vi "ArchViewer.vi"() -> ()   [LabVIEW 2010]
doc: "Use this template to create an application that executes until you click the Stop button. Unlike the Single Loop Application VI that uses polling, this VI uses the Event structure."
uses:
  <vilib>/addons/database/Connection.llb/DB Tools Open Connec (Path).vi
  <vilib>/addons/database/NI_Database_API.lvlib
panel:
  in  "save":bool
  out "Message":string
  out "ObjProp":string[][](table)
  in  "ViewMode":enum32{"Графики", "Тренды", "SQL"}(tab)=enum."Тренды"
  out "reason":string caption="Описание"
  in  "DateAndTime":u16(ring) caption="Дата и Время" items=["2010-03-20 19:57:10", "2010-03-20 19:58:10", "2010-03-20 19:59:11", "2010-03-20 20:00:11", "2010-03-20 20:01:12", "2010-03-20 20:02:12", "2010-03-20 20:03:13"]
  out "Waveform Graph":cluster{sgl, sgl, sgl[]}[](graph)
  in  "CurvesName":i32(ring) caption="Сигнал (Тип сигнала)" items=["Q(wt)max"=400301, "Q(wt)mean"=500301, "Q(R)"=300301, "I(R)"=100301, "N(Q)"=200301]
  out "XY Graph":cluster{timestamp[], sgl[]}(graph)
  in  "T final":timestamp caption="Конец интервала"
  in  "T start":timestamp caption="Начало"
  in  "SigName":u16(ring) caption="Сигнал" items=["In(Напряжение/Ток)"=302, "Out(Напряжение/Ток)"=301]
  in  "Numeric":i32 min=0 max=9
  in  "Execute":bool
  out "Data":string[][](table) caption="Данные"
  in  "Query":string caption="Запрос"
  in  "Tables":i32(listbox) caption="Таблицы"
  in  "Object":u16(ring) caption="Объект" items=["test1", "К-19 Тц", "Безымянный", "test2"]
  in  "stop":bool
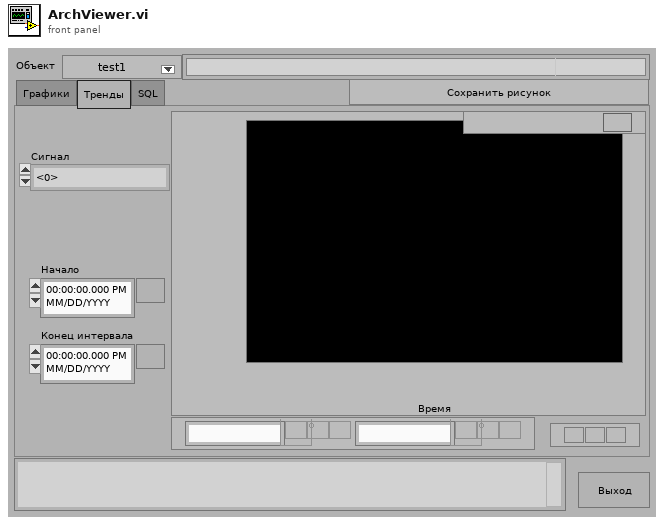
[diagram p1: front panel]
types:
  T1 = typedef "NI_Database_API.lvlib/Conn ObjectReference.ctl" = refnum<k1>
  T2 = cluster{"recordset data[0]":variant, "recordset data[1]":variant}
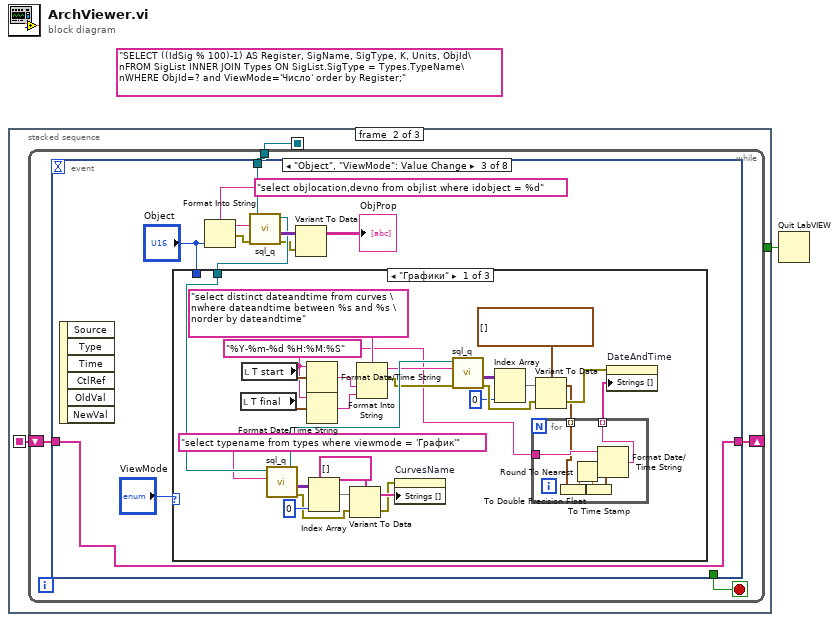
[diagram p0: block diagram]
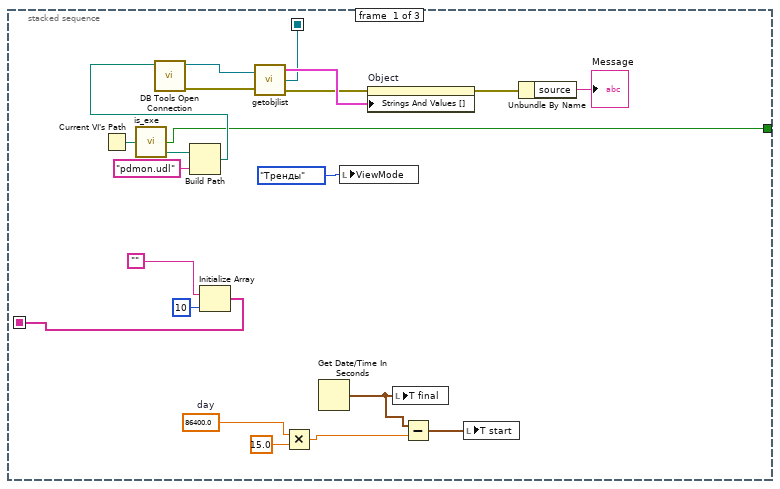
[diagram p2: hidden frame]
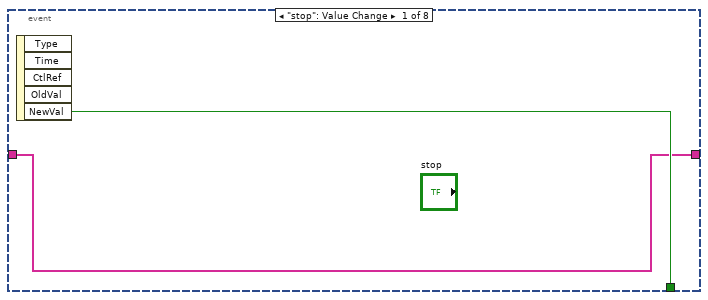
[diagram p3: hidden frame]
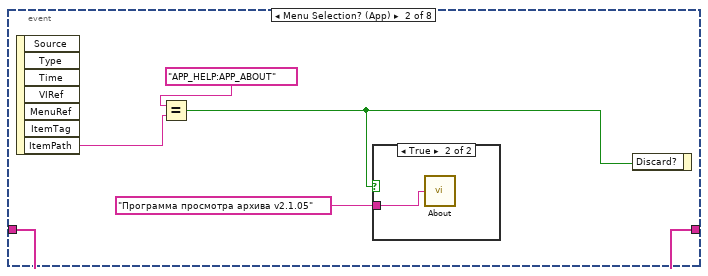
[diagram p4: hidden frame]
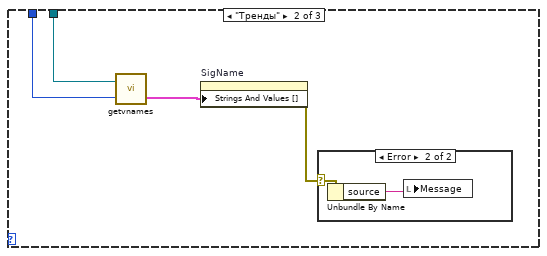
[diagram p6: hidden frame]
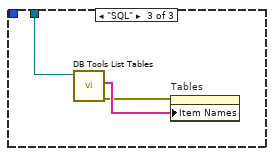
[diagram p8: hidden frame]
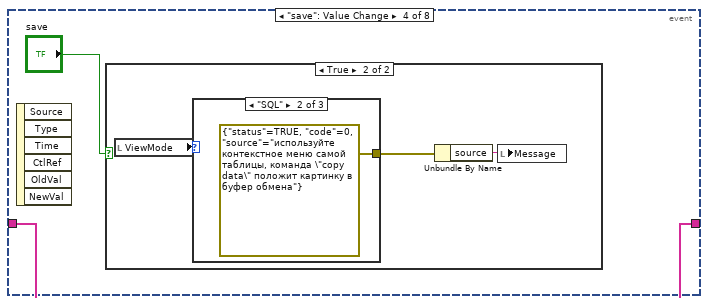
[diagram p9: hidden frame]
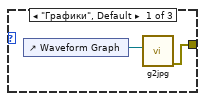
[diagram p11: hidden frame]
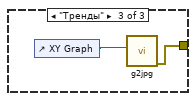
[diagram p12: hidden frame]
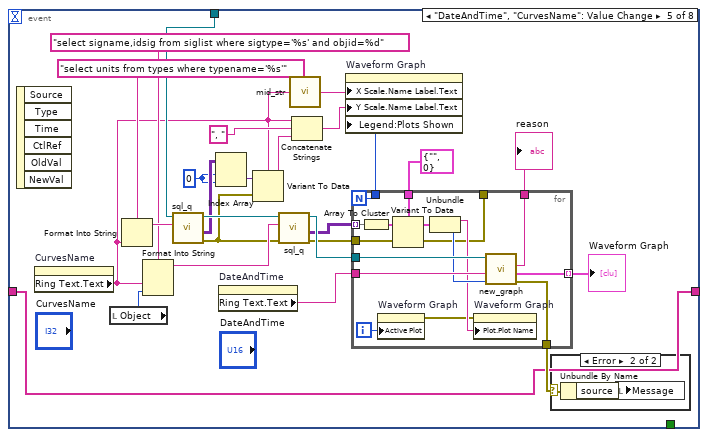
[diagram p13: hidden frame]
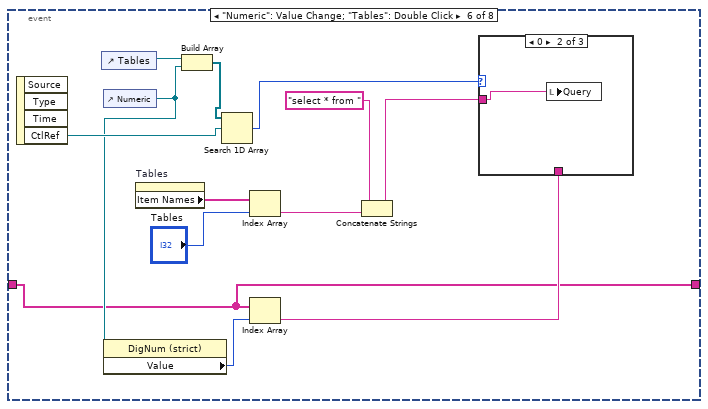
[diagram p15: hidden frame]
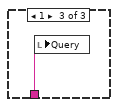
[diagram p17: hidden frame]
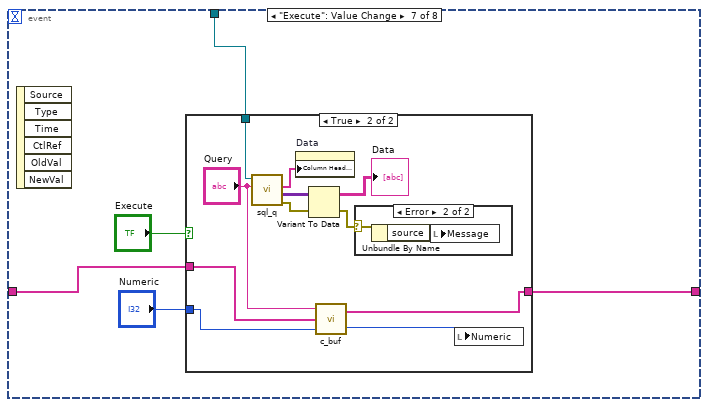
[diagram p18: hidden frame]
diagram:
  (unwired) "SELECT ((IdSig % 100)-1) AS Register, SigName, SigType, K, Units, ObjId\nFROM SigList INNER JOIN Types ON SigList.SigType = Types.TypeName\nWHERE ObjId=? and ViewMode='Число' order by Register;"
  n1 = stacked-sequence {
    seq-local: [w18 _ _] -> [_ w24 w189]
    seq-local: [w3 _ _] -> [_ w23 _]
    tunnel: [w2 _ _] -> w1
    frame #0 {
      w8 = 86400.0  # day
      n2 = Current VI's Path() -> (path=w14:path)
      n3 = call "is_exe.vi"("path"=w14) -> ("actual path"=w13:path, "exe?"=w2:bool)  [unwired: 2 in, 1 out]
      n4 = Build Path(base path=w13, name or relative path="pdmon.udl") -> (appended path=w11:path)
      n5 = call-poly <vilib>:"DB Tools Open Connection.vi"("connection information"=w11) -> ("error out"=w19:errorcluster, "connection reference"=w20:T1)  [unwired: 7 in]
      n6 = Initialize Array("", 10 ("dimension size")) -> (w3:string[])
      n7 = call "getobjlist.vi"("connection"=w20, "error in"=w19) -> ("StringsAndValues[]"=w22:cluster{"String":string, "Value":u16}[], "connection out"=w18:T1, "error out"=w21:errorcluster)
      n8 = Multiply(x=w8, y=15.0) -> (x*y=w7:dbl)
      n9 = Get Date/Time In Seconds() -> (seconds since 1Jan1904=w10:timestamp)
      n10 = local write "ViewMode"(enum32{"Графики", "Тренды", "SQL"}."Тренды" ("ViewMode")) -> ()
      n11 = property on="Object" class="Ring (strict)"(error in=w21, "Strings And Values []"=w22) -> (error out=w17:errorcluster)  [unwired: 1 in, 1 out]
      n12 = local write "T final"(w10) -> ()
      n13 = Subtract(x=w10, y=w7) -> (x-y=w9:timestamp)
      n14 = local write "T start"(w9) -> ()
      n15 = Unbundle By Name(w17) -> ("source"=→"Message":string)
    }
    frame #1 {
      n16 = while {
        tunnel: w24 -> [w27]
        shift-right: [w26] -> _
        shift-left: w23 -> [w25]
        stop <- w28 stop-if-true
        n17 = event shown="[2] \"Object\", \"ViewMode\": Value Change" {
          selector: _ -> [_ _ _ _ _ _ _ _]
          dyn-events: _ -> [_ _ _ _ _ _ _ _]
          timeout: _ -> [_ _ _ _ _ _ _ _]
          tunnel: [w30 _ _ _ _ _ _ _] -> w28
          tunnel: w27 -> [_ _ w43 _ w112 _ w162 w186]
          tunnel: [w29 w35 w37 w89 w99 w143 w159 w178] -> w26
          tunnel: w25 -> [w29 w35 w37 w89 w99 w143 w158 w178]
          event "stop": Value Change {
            n18 = event-data() -> ("NewVal"=w30:bool)  [unwired: 1 in, 4 out]
          }
          event Menu Selection? (App) {
            n19 = event-data() -> ("ItemPath"=w33:string)  [unwired: 1 in, 6 out]
            n20 = Equal?(x="APP_HELP:APP_ABOUT", y=w33) -> (x = y?=w32:bool)
            n21 = case shown="True" w32 {
              tunnel: "Программа просмотра архива v2.1.05" -> [_ w36]
              frame False {
              }
              frame True {
                n22 = call "About.vi"("Revision Number"=w36) -> ()
              }
            }
            n23 = event-data("Discard?"=w32) -> ()  [unwired: 1 in, 1 out]
          }
          event "Object", "ViewMode": Value Change {
            n24 = event-data() -> ()  [unwired: 1 in, 6 out]
            n25 = Format Into String(format string="select objlocation,devno from objlist where idobject = %d", "Object") -> (resulting string=w46:string, error out=w39:errorcluster)  [unwired: 2 in]
            n26 = call "sql_q.vi"("error in"=w39, "SQL query"=w46, "connect ref"=w43) -> ("error out"=w41:errorcluster, "recordset data"=w45:variant[][], "conn ref out"=w42:T1)  [unwired: 1 in, 1 out]
            n27 = case shown="\"Графики\"" "ViewMode" {
              tunnel: w42 -> [w73 w82 w88]
              tunnel: "Object" -> [_ w81 _]
              frame "Графики" {
                w49 = "%Y-%m-%d %H:%M:%S" ("time format string (%c)")
                n28 = local read "T final"() -> (w60:timestamp)
                n29 = local read "T start"() -> (w61:timestamp)
                n30 = call "sql_q.vi"("SQL query"="select typename from types where viewmode = 'График'", "connect ref"=w73) -> ("error out"=w66:errorcluster, "recordset data"=w71:variant[][], "conn ref out"=w55:T1)  [unwired: 2 in, 1 out]
                n31 = Format Date/Time String(time format string (%c)=w49, seconds (now)=w61) -> (date/time string=w63:string)  [unwired: 1 in]
                n32 = Format Date/Time String(time format string (%c)=w49, seconds (now)=w60) -> (date/time string=w64:string)  [unwired: 1 in]
                n33 = Index Array(array=w71, index (col)=0 ("disabled index (col)")) -> (element=w68:variant[])  [unwired: 1 in]
                n34 = Variant To Data(error in=w66, Variant=w68, type=string[] [] ("Strings []")) -> (error out=w65:errorcluster, data=w70:string[])
                n35 = Format Into String(format string="select distinct dateandtime from curves \nwhere dateandtime between %s and %s \norder by dateandtime", w63, w64) -> (resulting string=w54:string, error out=w53:errorcluster)  [unwired: 2 in]
                n36 = property on="CurvesName" class="Ring (strict)"(error in=w65, "Strings []"=w70) -> ()  [unwired: 1 in, 2 out]
                n37 = call "sql_q.vi"("error in"=w53, "SQL query"=w54, "connect ref"=w55) -> ("error out"=w59:errorcluster, "recordset data"=w56:variant[][])  [unwired: 1 in, 2 out]
                n38 = Index Array(array=w56, index (col)=0 ("disabled index (col)")) -> (element=w57:variant[])  [unwired: 1 in]
                n39 = Variant To Data(error in=w59, Variant=w57, type=timestamp[] [] ("Strings []")) -> (error out=w52:errorcluster, data=w51:timestamp[])
                n40 = for {
                  tunnel: w51 -> [w74] mode=indexing
                  tunnel: [w79] -> w50 mode=indexing
                  tunnel: w49 -> [w78]
                  n41 = To Double Precision Float(number=w74) -> (double precision float=w76:dbl)
                  n42 = Round To Nearest(number=w76) -> (nearest integer value=w75:dbl)
                  n43 = To Time Stamp(1:w75) -> (0:w77:timestamp)
                  n44 = Format Date/Time String(time format string (%c)=w78, seconds (now)=w77) -> (date/time string=w79:string)  [unwired: 1 in]
                }
                n45 = property on="DateAndTime" class="Ring (strict)"(error in=w52, "Strings []"=w50) -> ()  [unwired: 1 in, 2 out]
              }
              frame "Тренды" {
                n46 = call "getvnames.vi"("Object"=w81, "connection reference in"=w82) -> ("StringsAndValues[]"=w83:cluster{"String":string, "Value":u16}[])  [unwired: 1 out]
                n47 = property on="SigName" class="Ring (strict)"("Strings And Values []"=w83) -> (error out=w80:errorcluster)  [unwired: 2 in, 1 out]
                n48 = case shown="Error" w80 {
                  selector: w80 -> [_ w85]
                  frame No Error {
                  }
                  frame Error {
                    n49 = Unbundle By Name(w85) -> ("source"=w84:string)
                    n50 = local write "Message"(w84) -> ()
                  }
                }
              }
              frame "SQL" {
                n51 = call <vilib>:"DB Tools List Tables.vi"("connection reference"=w88) -> ("error out"=w86:errorcluster, "tables"=w87:string[])  [unwired: 4 in, 1 out]
                n52 = property on="Tables" class="LstBox (strict)"(error in=w86, "Item Names"=w87) -> ()  [unwired: 1 in, 2 out]
              }
            }
            n53 = Variant To Data(error in=w41, Variant=w45) -> (data=→"ObjProp":string[][])  [unwired: 1 in, 1 out]
          }
          event "save": Value Change {
            n54 = event-data() -> ()  [unwired: 1 in, 6 out]
            n55 = case shown="True" "save" {
              frame False {
              }
              frame True {
                n56 = local read "ViewMode"() -> (w93:enum32{"Графики", "Тренды", "SQL"})
                n57 = case shown="\"SQL\"" w93 {
                  tunnel: [w94 errorcluster {"status"=TRUE, "code"=0, "source"="используйте контекстное меню самой таблицы, команда \"copy data\" положит картинку в буфер обмена"} ("error out") w97] -> w92
                  frame "Графики", Default {
                    n58 = control-ref of="Waveform Graph"() -> (w95:refnum<vi>)
                    n59 = call "g2jpg.vi"("WG"=w95) -> ("error out"=w94:errorcluster)  [unwired: 5 in, 1 out]
                  }
                  frame "SQL" {
                  }
                  frame "Тренды" {
                    n60 = control-ref of="XY Graph"() -> (w98:refnum<vi>)
                    n61 = call "g2jpg.vi"("WG"=w98) -> ("error out"=w97:errorcluster)  [unwired: 5 in, 1 out]
                  }
                }
                n62 = Unbundle By Name(w92) -> ("source"=w91:string)
                n63 = local write "Message"(w91) -> ()
              }
            }
          }
          event "DateAndTime", "CurvesName": Value Change {
            w108 = 0
            n64 = event-data() -> ()  [unwired: 1 in, 6 out]
            n65 = property on="CurvesName" class="Ring (strict)"() -> ("Ring Text.Text"=w100:string)  [unwired: 2 in, 2 out]
            n66 = local read "Object"() -> (w120:u16)
            n67 = Format Into String(format string="select units from types where typename='%s'", w100) -> (resulting string=w113:string)  [unwired: 2 in, 1 out]
            n68 = Format Into String(format string="select signame,idsig from siglist where sigtype='%s' and objid=%d" ("regular expression (\"\")"), w100, w120) -> (resulting string=w121:string)  [unwired: 2 in, 1 out]
            n69 = call "sql_q.vi"("SQL query"=w113, "connect ref"=w112) -> ("error out"=w105:errorcluster, "recordset data"=w109:variant[][], "conn ref out"=w111:T1)  [unwired: 2 in, 1 out]
            n70 = Index Array(array=w109, index (row)=w108, index (col)=w108) -> (element=w107:variant)
            n71 = property on="DateAndTime" class="Ring (strict)"() -> ("Ring Text.Text"=w124:string)  [unwired: 2 in, 2 out]
            n72 = Variant To Data(error in=w105, Variant=w107, type=w100) -> (data=w104:string)  [unwired: 1 out]
            n73 = call "sql_q.vi"("error in"=w105, "SQL query"=w121, "connect ref"=w111) -> ("error out"=w110:errorcluster, "recordset data"=w118:variant[][], "conn ref out"=w119:T1)  [unwired: 1 in, 1 out]
            n74 = call "mid_str.vi"("String"=w100) -> ("mid substring"=w101:string)  [unwired: 4 in]
            n75 = Concatenate Strings(w100, ", ", w104) -> (w103:string)
            n76 = for {
              N -> [w127]
              tunnel: w124 -> [w140]
              tunnel: [w139] -> w123
              tunnel: [w138] -> w122
              tunnel: w119 -> [w137]
              tunnel: w118 -> [w136] mode=indexing
              tunnel: cluster{string, i32} {"", 0} -> [w135]
              tunnel: [w131] -> w116 mode=indexing
              tunnel: [w127] -> w115
              tunnel: w110 -> [w126]
              tunnel: [w125] -> _
              i -> [w130]
              n77 = Array To Cluster(array=w136) -> (cluster=w134:T2)
              n78 = property on="Waveform Graph" class="WFGraph (strict)"("Active Plot"=w130) -> (error out=w128:errorcluster)  [unwired: 2 in, 1 out]
              n79 = Variant To Data(error in=w126, Variant=w134, type=w135) -> (error out=w125:errorcluster, data=w133:cluster{string, i32})
              n80 = Unbundle(w133) -> (w129:string, w132:i32)
              n81 = property on="Waveform Graph" class="WFGraph (strict)"(error in=w128, "Plot.Plot Name"=w129) -> ()  [unwired: 1 in, 2 out]
              n82 = call "new_graph.vi"("CurvesId"=w132, "D&T"=w140, "connection ref"=w137) -> ("error out"=w139:errorcluster, "Waveform Graph"=w131:cluster{sgl, sgl, sgl[]}, "reason"=w138:string)  [unwired: 2 in]
            }
            "Waveform Graph" <- w116
            "reason" <- w122
            n83 = property on="Waveform Graph" class="WFGraph (strict)"("X Scale.Name Label.Text"=w101, "Y Scale.Name Label.Text"=w103, "Legend:Plots Shown"=w115) -> ()  [unwired: 2 in, 2 out]
            n84 = case shown="Error" w123 {
              selector: w123 -> [_ w142]
              frame No Error {
              }
              frame Error {
                n85 = Unbundle By Name(w142) -> ("source"=w141:string)
                n86 = local write "Message"(w141) -> ()
              }
            }
          }
          event "Numeric": Value Change; "Tables": Double Click {
            n87 = event-data() -> ("CtlRef"=w149:refnum<vi>)  [unwired: 1 in, 3 out]
            n88 = control-ref of="Tables"() -> (w151:refnum<vi>)
            n89 = control-ref of="Numeric"() -> (w145:refnum<vi>)
            n90 = property on="Property Node" class="DigNum (strict)"(reference=w145) -> ("Value"=w144:i32)  [unwired: 1 in, 2 out]
            n91 = property on="Tables" class="LstBox (strict)"() -> ("Item Names"=w155:string[])  [unwired: 2 in, 2 out]
            n92 = Build Array(w151, w145) -> (w150:refnum<vi>[])
            n93 = Search 1D Array(1D array=w150, element=w149) -> (index of element=w148:i32)  [unwired: 1 in]
            n94 = Index Array(array=w155, index="Tables") -> (element=w153:string)
            n95 = Index Array(array=w143, index=w144) -> (element=w146:string)
            n96 = Concatenate Strings("select * from " ("format string"), w153) -> (w147:string)
            n97 = case shown="0" w148 {
              tunnel: w147 -> [_ w156 _]
              tunnel: w146 -> [_ _ w157]
              frame -1, Default {
                # "do nothing"
              }
              frame 0 {
                n98 = local write "Query"(w156) -> ()
              }
              frame 1 {
                n99 = local write "Query"(w157) -> ()
              }
            }
          }
          event "Execute": Value Change {
            n100 = event-data() -> ()  [unwired: 1 in, 6 out]
            n101 = case shown="True" "Execute" {
              tunnel: w162 -> [_ w174]
              tunnel: "Numeric" -> [_ w167]
              tunnel: [w163 w168] -> w159
              tunnel: w158 -> [w163 w165]
              frame False {
              }
              frame True {
                n102 = call "sql_q.vi"("SQL query"="Query", "connect ref"=w174) -> ("error out"=w171:errorcluster, "recordset data"=w173:variant[][], "Columns"=w170:string[])  [unwired: 2 in, 1 out]
                n103 = property on="Data" class="Tbl (strict)"("Column Header Strings[]"=w170) -> ()  [unwired: 2 in, 2 out]
                n104 = Variant To Data(error in=w171, Variant=w173) -> (error out=w169:errorcluster, data=→"Data":string[][])  [unwired: 1 in]
                n105 = call "c_buf.vi"("Numeric 2"=w167, "Array"=w165, "Query"="Query") -> ("Numeric"=w166:i32, "Array 2"=w168:string[])
                n106 = case shown="Error" w169 {
                  selector: w169 -> [_ w176]
                  frame No Error {
                  }
                  frame Error {
                    n107 = Unbundle By Name(w176) -> ("source"=w175:string)
                    n108 = local write "Message"(w175) -> ()
                  }
                }
                n109 = local write "Numeric"(w166) -> ()
              }
            }
          }
          event "SigName", "T start", "T final": Value Change {
            n110 = event-data() -> ()  [unwired: 1 in, 6 out]
            n111 = property on="SigName" class="Ring (strict)"() -> (error out=w179:errorcluster, "Ring Text.Text"=w180:string)  [unwired: 2 in, 1 out]
            n112 = call "new_trend.vi"("T start"="T start", "SigId"="SigName", "T final"="T final", "connection ref"=w186) -> ("error out"=w185:errorcluster, "XY Graph"=→"XY Graph":cluster{timestamp[], sgl[]}, "units"=w177:string)  [unwired: 1 out]
            n113 = property on="XY Graph" class="XYGraph (strict)"(error in=w179, "Plot.Plot Name"=w180, "Y Scale.Name Label.Text"=w177) -> ()  [unwired: 1 in, 2 out]
            n114 = case shown="Error" w185 {
              selector: w185 -> [_ w188]
              frame No Error {
              }
              frame Error {
                n115 = Unbundle By Name(w188) -> ("source"=w187:string)
                n116 = local write "Message"(w187) -> ()
              }
            }
          }
        }
      }
    }
    frame #2 {
      n117 = call <vilib>:"DB Tools Close Connection.vi"("connection reference"=w189) -> ()  [unwired: 6 in, 1 out]
    }
  }
  n118 = Quit LabVIEW(quit? (T)=w1) -> ()
